vi "LakeShore336_Viewer.vi"() -> ()   [LabVIEW 2018]
uses:
  <instrlib>/Lake Shore 336/Public/Data/Sensor Data (Single Reading).vi
  <instrlib>/Lake Shore 336/Lake Shore 336.lvlib
panel:
  in  "stop":bool
  out "Temp vs Vg : XYGraph":cluster{"Y":dbl[], "Y":dbl[]}[](graph)
  out "Temp vs Vg : TimeGraph":cluster{i32, "Sensor Data":dbl}[](graph)
  in  "Data Source (0:Kelvin)":u16(ring) items=["Kelvin", "Celsius", "Sensor Units"]
  in  "Input (0:A)":u16(ring) items=["A", "B", "C", "D"]
  in  "Serial Configuration 2":T1={"Baud Rate"=57600, "Parity"=1, "Data Bits"=7, "Stop Bits"=10, "Flow Control"=0} {"Flow Control" items=["None", "XON/XOFF", "RTS/CTS", "XON/XOFF & RTS/CTS", "DTR/DSR", "XON/XOFF & DTR/DSR"]; "Stop Bits" items=["1.0"=10, "1.5"=15, "2.0"=20]; "Data Bits" items=["7"=7, "8"=8]; "Parity" items=["None", "Odd", "Even", "Mark", "Space"]; "Baud Rate" items=["300"=300, "600"=600, "1200"=1200, "2400"=2400, "4800"=4800, "9600"=9600, "19200"=19200, "38400"=38400, "57600"=57600]}
  in  "LakeShore 336 esource name":refnum<visa-resource-name>
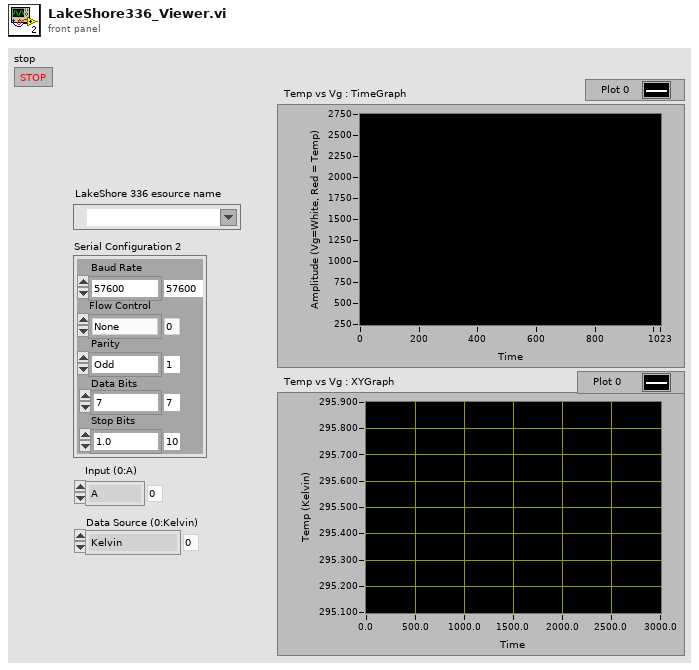
[diagram p1: front panel]
types:
  T1 = cluster{"Baud Rate":u32, "Parity":u16, "Data Bits":u16, "Stop Bits":u16, "Flow Control":u16}
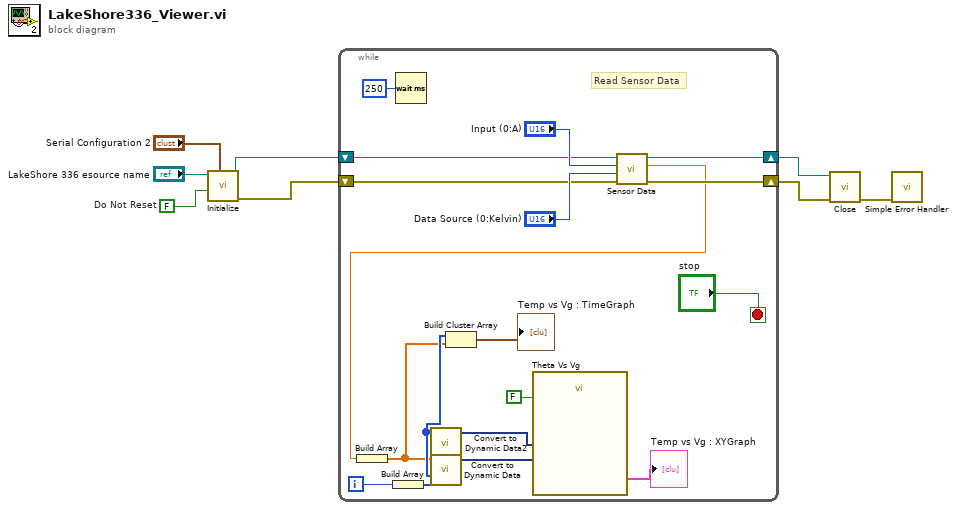
[diagram p0: block diagram]
diagram:
  w6 = FALSE  # Do Not Reset
  n1 = call <instrlib>:"Initialize.vi"("Serial Configuration"="Serial Configuration 2", "Reset (True)"=w6, "VISA resource name"="LakeShore 336 esource name") -> ("error out"=w1:errorcluster, "VISA resource name out"=w2:refnum<visa-resource-name>)  [unwired: 7 in]
  n2 = while {
    shift-right: [w23] -> w4
    shift-left: w2 -> [w21]
    shift-right: [w22] -> w3
    shift-left: w1 -> [w20]
    i -> [w13]
    stop <- "stop" stop-if-true
    # "Read Sensor Data"
    n3 = Build Array(w13) -> (w11:i32[])
    n4 = Wait (ms)(milliseconds to wait=u32 250) -> ()  [unwired: 1 out]
    n5 = call "Convert to Dynamic Data2"("Array"=w11) -> ("Dynamic Data Type"=w12:dynamicdata)  [unwired: 3 in]
    n6 = call-poly <instrlib>:"Sensor Data.vi"("error in (no error)"=w20, "Data Source (0:Kelvin)"="Data Source (0:Kelvin)", "Input (0:A)"="Input (0:A)", "VISA resource name"=w21) -> ("error out"=w22:errorcluster, "Sensor Data"=w15:dbl, "VISA resource name out"=w23:refnum<visa-resource-name>)  [unwired: 5 in]
    n7 = Build Array(w15) -> (w10:dbl[])
    n8 = call "Convert to Dynamic Data"("Array"=w10) -> ("Dynamic Data Type"=w14:dynamicdata)  [unwired: 3 in]
    n9 = Build Cluster Array(w11, w10) -> (→"Temp vs Vg : TimeGraph":cluster{i32, "Sensor Data":dbl}[])
    n10 = call "Theta Vs Vg"("Reset"=FALSE, "Y Input"=w14, "X Input"=w12) -> ("XY Graph"=→"Temp vs Vg : XYGraph":cluster{"X":dbl[], "Y":dbl[]}[])  [unwired: 7 in, 1 out]
  }
  n11 = call <instrlib>:"Close.vi"("error in (no error)"=w3, "VISA resource name"=w4) -> ("error out"=w7:errorcluster)  [unwired: 9 in]
  n12 = call <vilib>:"Simple Error Handler.vi"("error in (no error)"=w7) -> ()  [unwired: 4 in, 5 out]
